vi "Deconstruct PDU.vi"(8 "error in":errorcluster, 11 "SMSD data unit in":refnum<class "SMSD Data Unit.lvclass">) -> (0 "error out":errorcluster, 2 "DATA":u8[](array[numeric]), 3 "CMD_TYPE":T1(ring))   [LabVIEW 2021, in "SMSD Data Unit.lvclass"]
uses:
  SMSD Data Unit.lvclass
  SMSD Data Unit.lvclass/SMSD Data Unit.ctl
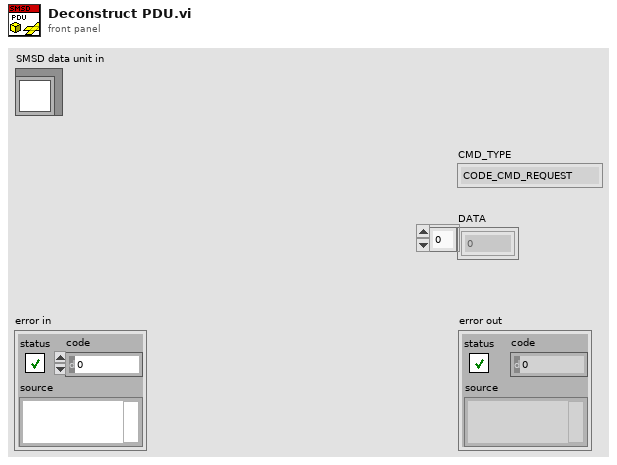
[diagram p1: front panel]
types:
  T1 = enum8{"CODE_CMD_REQUEST", "CODE_CMD_RESPONSE", "CODE_CMD_POWERSTEP01", "CODE_CMD_POWERSTEP01_W_MEM0", "CODE_CMD_POWERSTEP01_W_MEM1", "CODE_CMD_POWERSTEP01_W_MEM2", "CODE_CMD_POWERSTEP01_W_MEM3", "CODE_CMD_POWERSTEP01_R_MEM0", "CODE_CMD_POWERSTEP01_R_MEM1", "CODE_CMD_POWERSTEP01_R_MEM2", "CODE_CMD_POWERSTEP01_R_MEM3", "CODE_CMD_CONFIG_SET", "CODE_CMD_CONFIG_GET", "CODE_CMD_PASSWORD_SET", "CODE_CMD_ERROR_GET"}
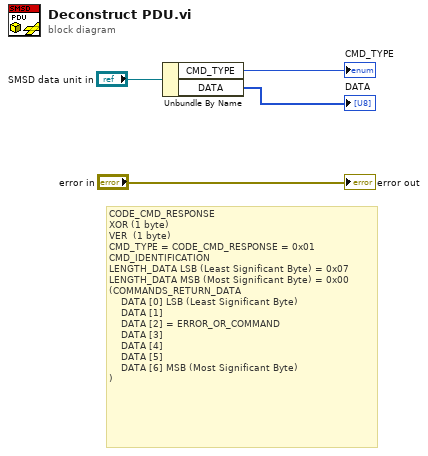
[diagram p0: block diagram]
diagram:
  # "CODE_CMD_RESPONSE\nXOR (1 byte)\nVER  (1 byte)\nCMD_TYPE = CODE_CMD_RESPONSE = 0x01\nCMD_IDENTIFICATION\nLENGTH_DATA LSB (Least Significant Byte) = 0x07\nLENGTH_DATA MSB (Most Significant Byte) = 0x00\n(COMMANDS_RETURN_DATA\n    DATA [0] LSB (Least Significant Byte)\n    DATA [1]\n    DATA [2] = ERROR_OR_COMMAND\n    DATA [3]\n    DATA [4]\n    DATA [5]\n    DATA [6] MSB (Most Significant Byte)\n)"
  n1 = Unbundle By Name("SMSD data unit in") -> ("CMD_TYPE"=→"CMD_TYPE":T1, "DATA"=→"DATA":u8[])
  "error out" <- "error in"
